vi "Test Report Contain Broken Error Type.vi"(8 "error in (no error)":errorcluster, 11 "XML Report Test in":refnum<class "XML Report Test.lvclass">) -> (0 "error out":errorcluster, 3 "XML Report Test out":refnum<class "XML Report Test.lvclass">)   [LabVIEW 2020, in "XML Report Test.lvclass"]
uses:
  XML Report Test.lvclass
  XML Report Test.lvclass/XML Report Test.ctl
  source/Plugins/XML Report/XML Report.lvclass
  source/Core/Result/Type.ctl
  source/Core/Result/Result.lvlib
  source/Core/Result/Status.ctl
  source/Core/Result/Result.ctl
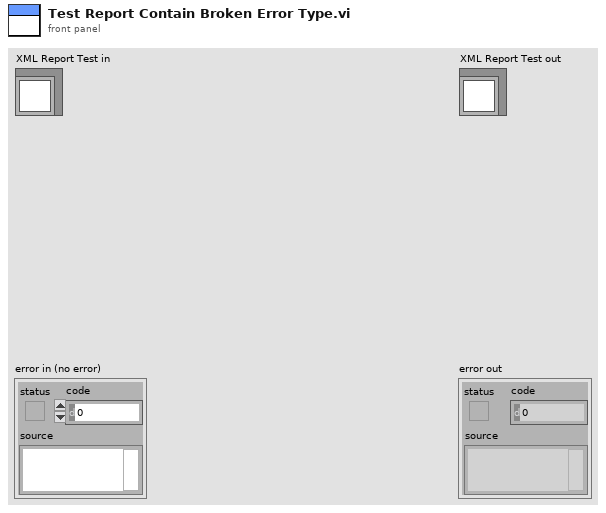
[diagram p1: front panel]
types:
  T1 = typedef "Result.lvlib/Result.ctl" = cluster{"Name":string, "Description":string, "Status":T2, "Result Type":T3, "Execution Time":dbl, "Data":cluster{"Expected":variant, "Actual":variant, "Delta":variant}}
  T2 = typedef "Result.lvlib/Status.ctl" = enum16{"", "Passed", "Failed", "Error", "Skipped", "Setup Error", "Broken", "Teardown Error"}
  T3 = typedef "Result.lvlib/Type.ctl" = enum16{"Test Case", "Test Suite", "Test Run", "Pass", "Fail", "Skip", "Pass if", "Fail if", "Pass if Error", "Fail if Error", "Pass if Equal", "Fail if Equal"}
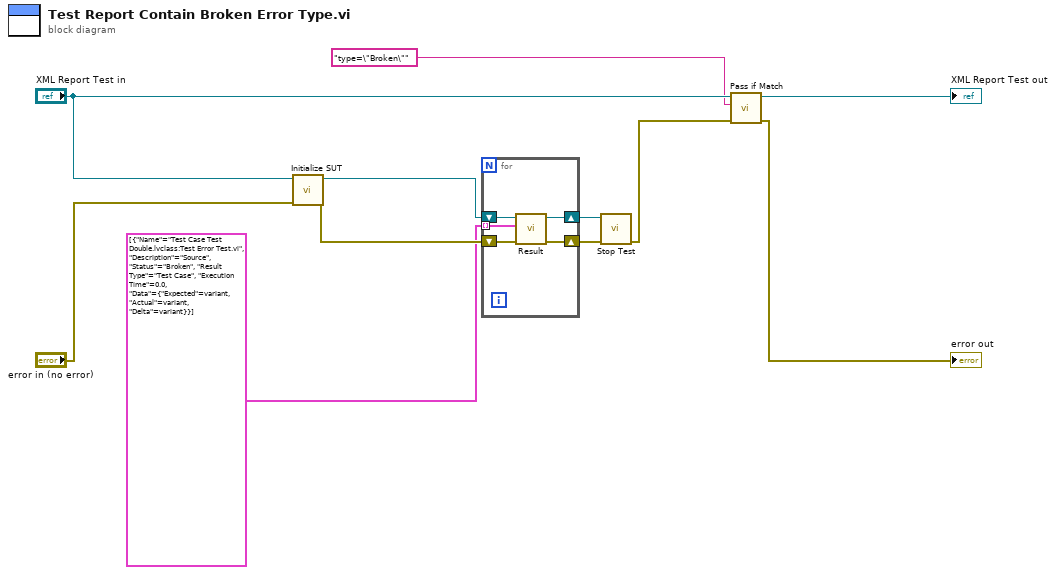
[diagram p0: block diagram]
diagram:
  n1 = call "Initialize SUT.vi"("error in (no error)"="error in (no error)", "XML Report Test in"="XML Report Test in") -> ("error out"=w11:errorcluster, "XML Report out"=w3:refnum<class "XML Report.lvclass">)  [unwired: 8 in]
  n2 = for {
    tunnel: T1[] [{"Name"="Test Case Test Double.lvclass:Test Error Test.vi", "Description"="Source", "Status"=enum."Broken", "Result Type"=enum."Test Case", "Execution Time"=0.0, "Data"={"Expected"=variant, "Actual"=variant, "Delta"=variant}}] ("Data") -> [w12] mode=indexing
    shift-right: [w15] -> w4
    shift-left: w11 -> [w16]
    shift-right: [w13] -> w2
    shift-left: w3 -> [w14]
    n3 = call-dynamic "Result.vi"("error in (no error)"=w16, "Result"=w12, "XML Report In"=w14) -> ("error out"=w15:errorcluster, "XML Report Out"=w13:refnum<class "XML Report.lvclass">)  [unwired: 7 in]
  }
  n4 = call-dynamic "Stop Test.vi"("error in (no error)"=w4, "XML Report In"=w2) -> ("error out"=w7:errorcluster)  [unwired: 8 in, 1 out]
  n5 = call "Pass if Match.vi"("error in (no error)"=w7, "regular expression"="type=\"Broken\"", "XML Report Test in"="XML Report Test in") -> ("error out"=→"error out":errorcluster, "XML Report Test out"=→"XML Report Test out":refnum<class "XML Report Test.lvclass">)  [unwired: 6 in, 1 out]
